vi "Fiducial Parameters.vi"(8 "error in (no error)":errorcluster, 10 "Fiducial Type":string, 11 "FlexWorktable in":refnum<class "FlexWorktable.lvclass">) -> (0 "error out":errorcluster, 1 "Fiducial Parameters":variant, 2 "Fiducial Method":string, 3 "FlexWorktable out":refnum<class "FlexWorktable.lvclass">, 4 "debug enable":bool)   [LabVIEW 2017, in "FlexWorktable.lvclass"]
uses:
  FlexWorktable.lvclass
  External/Vision/find_circles parameters.ctl
  External/Vision/find_patches parameters.ctl
  External/Vision/find_rects_parameters.ctl
  External/Vision/Vision.lvlib
panel:
  in  "find_rects parameters":T1
  in  "find_patches parameters":T2
  in  "find_circles parameters":T3
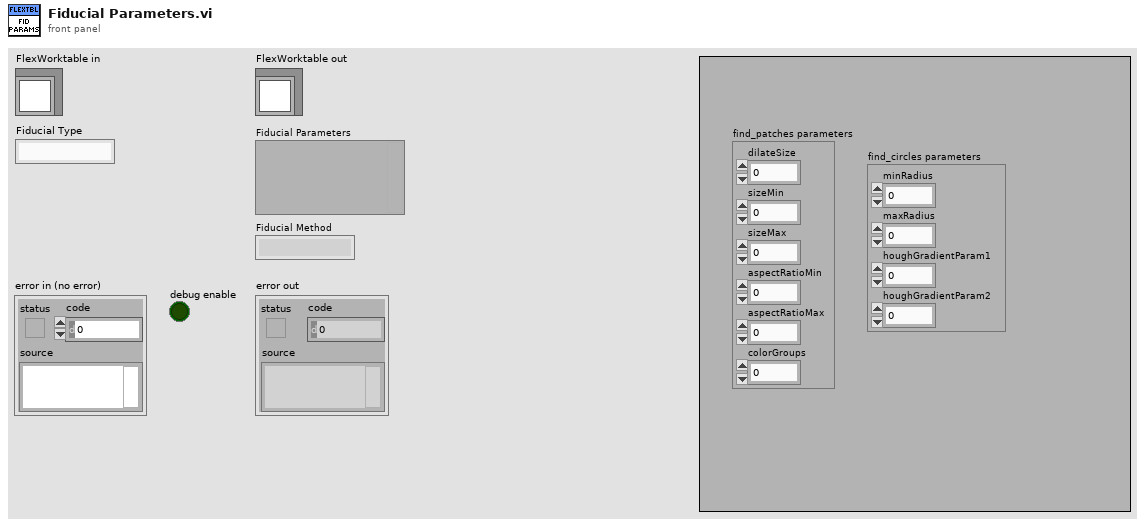
[diagram p1: front panel]
types:
  T1 = typedef "Vision.lvlib/find_rects_parameters.ctl" = cluster{"nominalWidth":sgl, "nominalHeight":sgl, "tolerance":sgl, "pointSelect":sgl, "allowRotation":bool}
  T2 = typedef "Vision.lvlib/find_patches parameters.ctl" = cluster{"dilateSize":i32, "sizeMin":sgl, "sizeMax":sgl, "aspectRatioMin":sgl, "aspectRatioMax":sgl, "colorGroups":i32}
  T3 = typedef "Vision.lvlib/find_circles parameters.ctl" = cluster{"minRadius":sgl, "maxRadius":sgl, "houghGradientParam1":i32, "houghGradientParam2":i32}
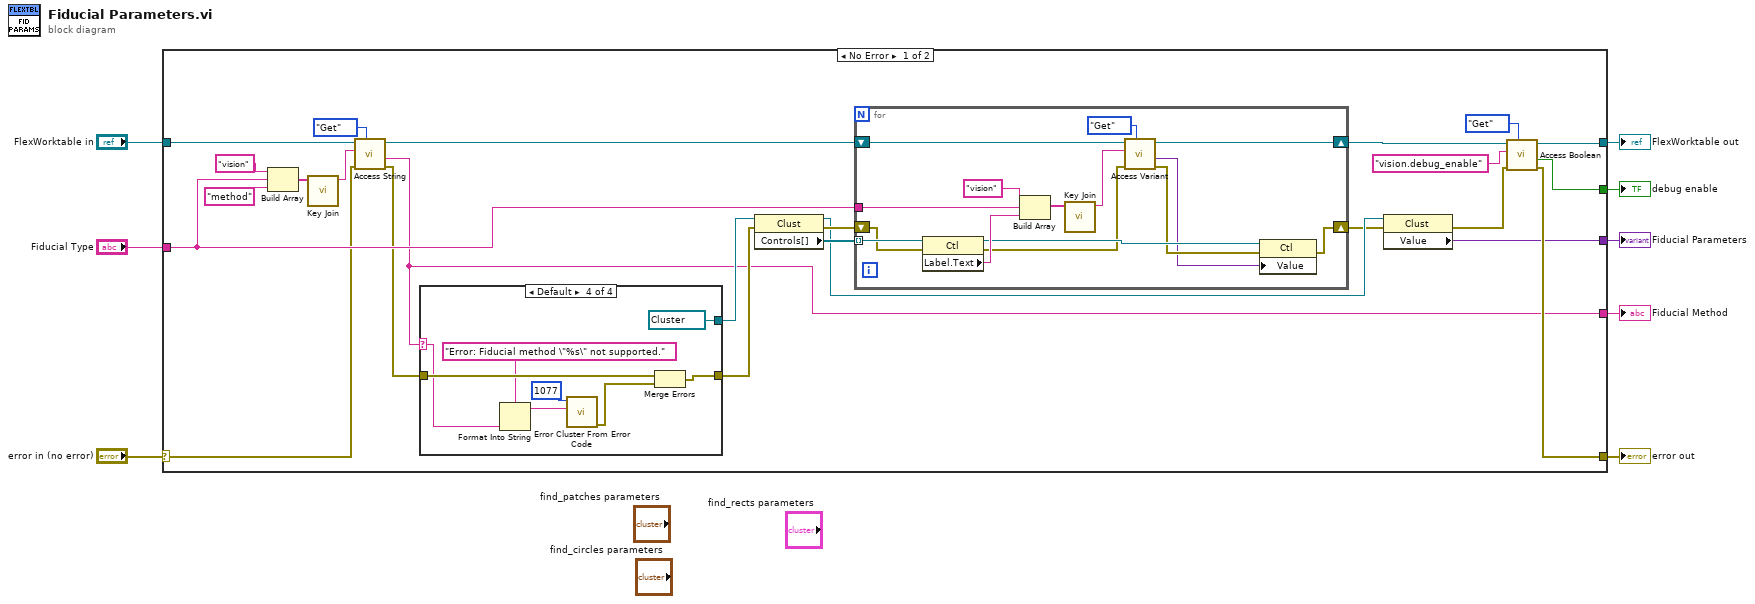
[diagram p0: block diagram]
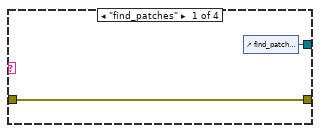
[diagram p2: hidden frame]
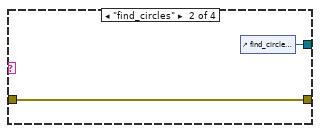
[diagram p3: hidden frame]
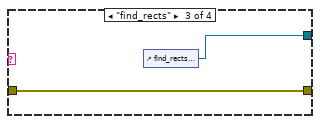
[diagram p4: hidden frame]
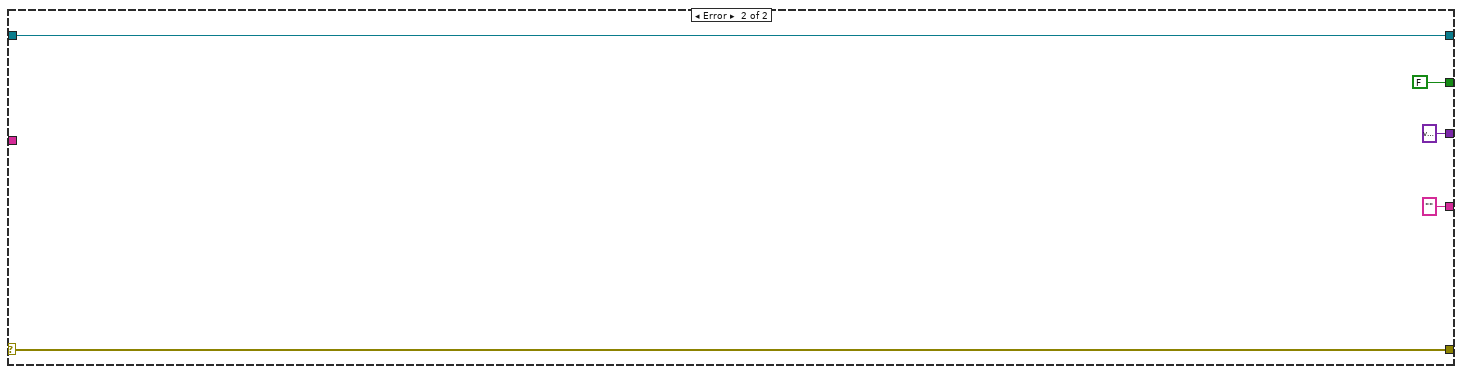
[diagram p5: hidden frame]
diagram:
  n1 = case shown="No Error" "error in (no error)" {
    selector: "error in (no error)" -> [w20 w67]
    tunnel: [w28 w67] -> w7
    tunnel: [w32 w66] -> w5
    tunnel: "FlexWorktable in" -> [w27 w66]
    tunnel: "Fiducial Type" -> [w24 _]
    tunnel: [w13 variant ("Value")] -> w2
    tunnel: [w29 FALSE ("Value out")] -> w3
    tunnel: [w9 "" ("Value out")] -> w1
    frame No Error {
      n2 = Build Array("vision", w24, "method" ("element")) -> (w26:string[])
      n3 = call "Key Join.vi"("Key Elements"=w26) -> ("Key"=w22:string)  [unwired: 10 in]
      n4 = call-dynamic "Access String.vi"("Get/Set"=enum16{"Get", "Set"}."Get", "error in (no error)"=w20, "Key"=w22, "FlexWorktable in"=w27) -> ("error out"=w11:errorcluster, "Value out"=w9:string, "FlexWorktable out"=w19:refnum<class "FlexWorktable.lvclass">)  [unwired: 5 in]
      n5 = case shown="Default" w9 {
        selector: w9 -> [_ _ _ w41]
        tunnel: [w35 w37 w39 refnum<vi> refnum ("find_circles parameters")] -> w18
        tunnel: w11 -> [w34 w36 w38 w45]
        tunnel: [w34 w36 w38 w44] -> w10
        frame "find_patches" {
          n6 = control-ref of="find_patches parameters"() -> (w35:refnum<vi>)
        }
        frame "find_circles" {
          n7 = control-ref of="find_circles parameters"() -> (w37:refnum<vi>)
        }
        frame "find_rects" {
          n8 = control-ref of="find_rects parameters"() -> (w39:refnum<vi>)
        }
        frame Default {
          n9 = Format Into String(format string="Error: Fiducial method \"%s\" not supported.", w41) -> (resulting string=w40:string)  [unwired: 2 in, 1 out]
          n10 = call <vilib>:"Error Cluster From Error Code.vi"("error message (\"\")"=w40, "error code (0)"=1077) -> ("error out"=w46:errorcluster)  [unwired: 7 in]
          n11 = Merge Errors(w45, w46) -> (w44:errorcluster)
        }
      }
      n12 = property class="Clust"(reference=w18, error in=w10) -> (reference out=w15:refnum<vi>, error out=w16:errorcluster, "Controls[]"=w17:refnum<vi>[])
      n13 = for {
        tunnel: w24 -> [w62]
        shift-right: [w48] -> w33
        shift-left: w19 -> [w53]
        shift-right: [w55] -> w14
        shift-left: w16 -> [w56]
        tunnel: w17 -> [w59] mode=indexing
        n14 = property class="Ctl"(reference=w59, error in=w56) -> (reference out=w57:refnum<vi>, error out=w51:errorcluster, "Label.Text"=w58:string)
        n15 = Build Array("vision", w62, w58) -> (w60:string[])
        n16 = call "Key Join.vi"("Key Elements"=w60) -> ("Key"=w54:string)  [unwired: 10 in]
        n17 = call-dynamic "Access Variant.vi"("Get/Set"=enum16{"Get", "Set"}."Get", "error in (no error)"=w51, "Key"=w54, "FlexWorktable in"=w53) -> ("error out"=w50:errorcluster, "Value out"=w49:variant, "FlexWorktable out"=w48:refnum<class "FlexWorktable.lvclass">)  [unwired: 5 in]
        n18 = property class="Ctl"(reference=w57, error in=w50, "Value"=w49) -> (error out=w55:errorcluster)  [unwired: 1 out]
      }
      n19 = property class="Clust"(reference=w15, error in=w14) -> (error out=w12:errorcluster, "Value"=w13:variant)  [unwired: 1 out]
      n20 = call-dynamic "Access Boolean.vi"("Get/Set"=enum16{"Get", "Set"}."Get", "error in (no error)"=w12, "Key"="vision.debug_enable", "FlexWorktable in"=w33) -> ("error out"=w28:errorcluster, "Value out"=w29:bool, "FlexWorktable out"=w32:refnum<class "FlexWorktable.lvclass">)  [unwired: 5 in]
    }
    frame Error {
    }
  }
  "error out" <- w7
  "FlexWorktable out" <- w5
  "debug enable" <- w3
  "Fiducial Parameters" <- w2
  "Fiducial Method" <- w1
